vi "Write Config.vi"(8 "error in (no error)":errorcluster, 9 "Re-Init?":bool, 10 "ICM File In":path, 11 "No-op Parser in":refnum<class "No-op Parser.lvclass">) -> (0 "error out":errorcluster, 3 "No-op Parser out":refnum<class "No-op Parser.lvclass">)   [LabVIEW 2015, in "No-op Parser.lvclass"]
doc: "No-op Parser.lvclass:Write Config.vi\n\nThis VI writes the configuration parameters for the No-op Parser class.\n\nInstrument Communication Module Version 1.0\nJanuary, 2018 Original Code Consulting David Thomson\n www.originalcode.com"
uses:
  No-op Parser.lvclass
  No-op Parser.lvclass/No-op Parser.ctl
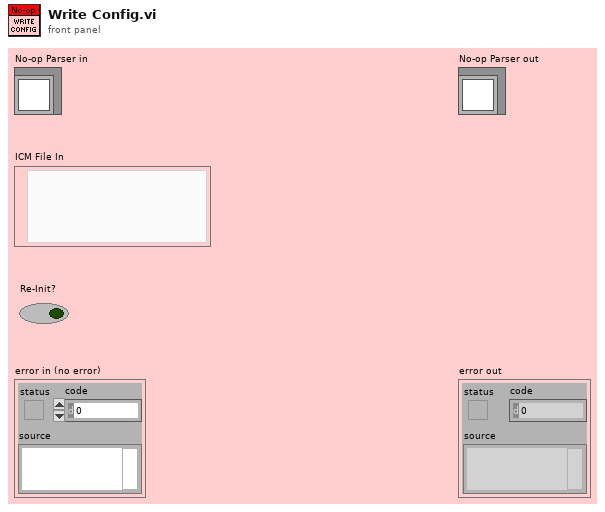
[diagram p1: front panel]
types:
  T1 = typedef "No-op Parser Config.ctl" = cluster{"Channels":string[], "Enabled":bool[]}
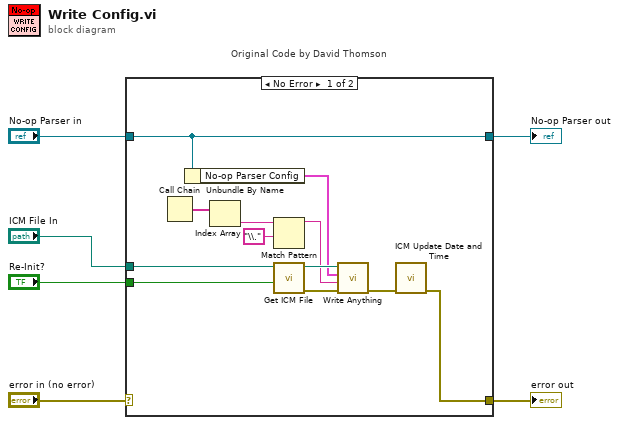
[diagram p0: block diagram]
diagram:
  n1 = case "Original Code by David Thomson" shown="No Error" "error in (no error)" {
    selector: "error in (no error)" -> [_ w20]
    tunnel: [w7 w20] -> w3
    tunnel: [w15 w19] -> w4
    tunnel: "No-op Parser in" -> [w15 w19]
    tunnel: "ICM File In" -> [w10 _]
    tunnel: "Re-Init?" -> [w9 _]
    frame No Error {
      n2 = Call Chain() -> (call chain=w17:string[])
      n3 = Unbundle By Name(w15) -> ("No-op Parser Config"=w11:T1)
      n4 = Index Array(array=w17) -> (element=w16:string)  [unwired: 1 in]
      n5 = Match Pattern(string=w16, regular expression="\\.") -> (before substring=w12:string)  [unwired: 1 in, 3 out]
      n6 = call "Get ICM File.vi"("Re-Init?"=w9, "ICM File In"=w10) -> ("error out"=w14:errorcluster, "ICM File"=w13:path)  [unwired: 8 in]
      n7 = call "Write Anything.vi"("Error In"=w14, "Section Name (Name of \"Anything\")"=w12, "Anything"=w11, "Path (dialog)"=w13) -> ("Error Out"=w8:errorcluster)  [unwired: 7 in]
      n8 = call "ICM Update Date and Time.vi"("error in (no error)"=w8) -> ("error out"=w7:errorcluster)  [unwired: 9 in, 1 out]
    }
    frame Error {
    }
  }
  "error out" <- w3
  "No-op Parser out" <- w4
